vi "svx_Orbit Direction.vi"(5 "revolutions":dbl=1.0 format="%.2f", 6 "shaft rotating direction":u16, 7 "actual samples/rev":dbl=64.0 format="%.2f", 10 "orbit plot Y":dbl[](array[numeric]), 11 "orbit plot X":dbl[](array[numeric])) -> (3 "orbit precession direction":u16(ring) items=["forward", "backward"])   [LabVIEW 2017, in "SVX Orbit.xctl"]
uses:
  <vilib>/addons/_XControls/Orbit Plot/SVX Orbit.xctl
  <vilib>/Analysis/1siggen.llb/Ramp Pattern by Samples.vi
  <vilib>/Analysis/NI_AALPro.lvlib
  <vilib>/Analysis/NI_AALBase.lvlib
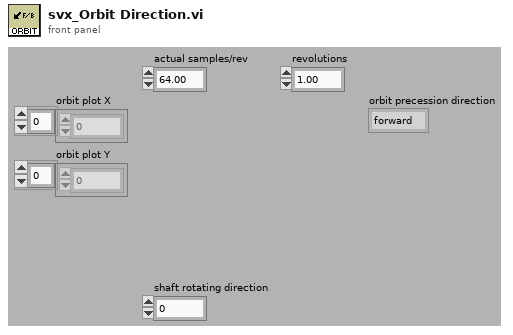
[diagram p1: front panel]
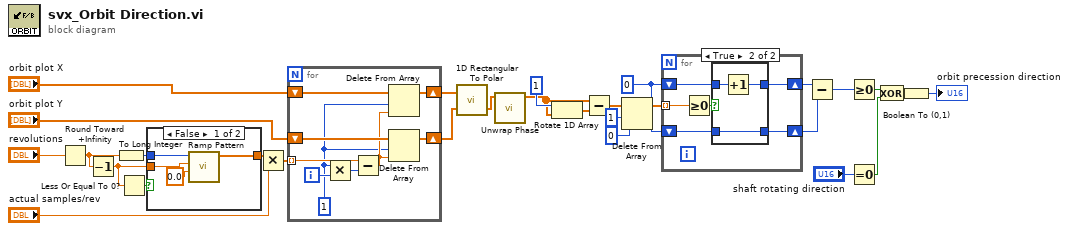
[diagram p0: block diagram]
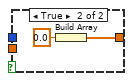
[diagram p2: hidden frame]
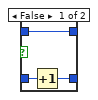
[diagram p3: hidden frame]
diagram:
  w11 = 0
  n1 = Round Toward +Infinity(x="revolutions") -> (ceil(x): smallest int >= x=w2:dbl)
  n2 = Decrement(x=w2) -> (x-1=w3:dbl)
  n3 = To Long Integer(number=w2) -> (32bit integer=w1:i32)
  n4 = Less Or Equal To 0?(x=w3) -> (x <= 0?=w4:bool)
  n5 = case shown="False" w4 {
    tunnel: w1 -> [w32 _]
    tunnel: w3 -> [w31 _]
    tunnel: [w30 w35] -> w10
    frame False {
      n6 = call-poly <vilib>:"Ramp Pattern.vi"("start"=0.0, "end"=w31, "samples"=w32) -> ("Ramp Pattern"=w30:dbl[])  [unwired: 7 in, 1 out]
    }
    frame True {
      n7 = Build Array(0.0 ("element")) -> (w35:dbl[])
    }
  }
  n8 = Multiply(x=w10, y="actual samples/rev") -> (x*y=w9:dbl[])
  n9 = for {
    shift-right: [w43] -> w8
    shift-left: "orbit plot X" -> [w44]
    tunnel: w9 -> [w42] mode=indexing
    shift-right: [w38] -> w7
    shift-left: "orbit plot Y" -> [w39]
    i -> [w41]
    w36 = 1 ("length")
    n10 = Multiply(x=w36, y=w41) -> (x*y=w40:i32)
    n11 = Subtract(x=w42, y=w40) -> (x-y=w37:dbl)
    n12 = Delete From Array(array=w44, length=w36, index=w37) -> (array with subset deleted=w43:dbl[])  [unwired: 1 out]
    n13 = Delete From Array(array=w39, length=w36, index=w37) -> (array with subset deleted=w38:dbl[])  [unwired: 1 out]
  }
  n14 = call <vilib>:"1D Rectangular To Polar.vi"("X"=w8, "Y"=w7) -> ("Phase"=w12:dbl[])  [unwired: 2 out]
  n15 = call <vilib>:"Unwrap Phase.vi"("Phase"=w12) -> ("Unwrapped Phase"=w14:dbl[])  [unwired: 9 in, 1 out]
  n16 = Rotate 1D Array(1:w14, 2:1 ("n")) -> (0:w16:dbl[])
  n17 = Subtract(x=w14, y=w16) -> (x-y=w17:dbl[])
  n18 = Delete From Array(array=w17, length=1, index=0) -> (array with subset deleted=w13:dbl[])  [unwired: 1 out]
  n19 = for {
    tunnel: w13 -> [w50] mode=indexing
    shift-right: [w46] -> w6
    shift-left: w11 -> [w48]
    shift-right: [w45] -> w5
    shift-left: w11 -> [w47]
    n20 = Greater Or Equal To 0?(x=w50) -> (x >= 0?=w49:bool)
    n21 = case shown="True" w49 {
      tunnel: w48 -> [w53 w56]
      tunnel: w47 -> [w52 w54]
      tunnel: [w53 w55] -> w46
      tunnel: [w51 w54] -> w45
      frame False {
        n22 = Increment(x=w52) -> (x+1=w51:i32)
      }
      frame True {
        n23 = Increment(x=w56) -> (x+1=w55:i32)
      }
    }
  }
  n24 = Subtract(x=w6, y=w5) -> (x-y=w20:i32)
  n25 = Greater Or Equal To 0?(x=w20) -> (x >= 0?=w22:bool)
  n26 = Equal To 0?(x="shaft rotating direction") -> (x = 0?=w23:bool)
  n27 = Exclusive Or(1:w23, 2:w22) -> (0:w24:bool)
  n28 = Boolean To (0,1)(Boolean=w24) -> (0, 1=→"orbit precession direction":i16)
